vi "ProgramDevice.vi"(1 "Firmware file":path) -> ()   [LabVIEW 2010]
panel:
  out "Array 4":u32[](array[numeric])
  out "Array 3":u32[][](array[numeric])
  out "Array 2":T1(array[cluster])
  out "Array":i32[][](array[numeric])
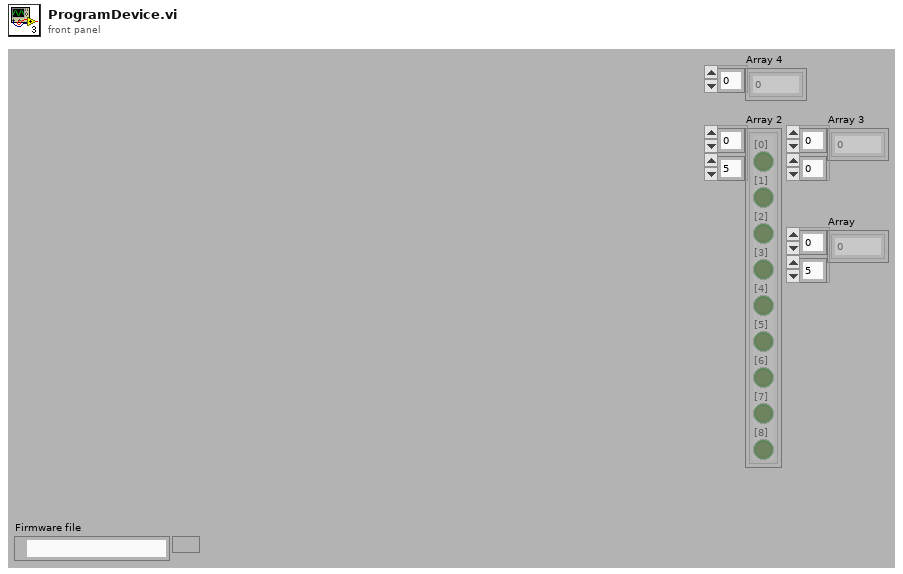
[diagram p1: front panel]
types:
  T1 = cluster{"[0]":bool, "[1]":bool, "[2]":bool, "[3]":bool, "[4]":bool, "[5]":bool, "[6]":bool, "[7]":bool, "[8]":bool}[][]
  T2 = cluster{"Clock Out MSB First":bool, "Clock Out On Positive Edge":bool}
  T3 = cluster{"Clock Pin State":bool, "Data Out Pin State":bool, "Chip Select Pin State":bool, "Chip Select Pin":u16}
  T4 = typedef "SpiDevice.ctl" = cluster{"Name":string, "Channel":string, "Location ID":u32, "Handle":u32}
  T5 = cluster{"Pin 1 State":bool, "Pin 1 Active State":bool, "Pin 2 State":bool, "Pin 2 Active State":bool, "Pin 3 State":bool, "Pin 3 Active State":bool, "Pin 4 State":bool, "Pin 4 Active State":bool, "Pin 5 State":bool, "Pin 5 Active State":bool, "Pin 6 State":bool, "Pin 6 Active State":bool, "Pin 7 State":bool, "Pin 7 Active State":bool, "Pin 8 State":bool, "Pin 8 Active State":bool}
  T6 = cluster{"Wait Data Write Complete":bool, "Wait Data Write Pin":u16, "Data Write Complete State":bool, "Data Write Timeout (ms)":u32}
  T7 = cluster{"[0]":bool, "[1]":bool, "[2]":bool, "[3]":bool, "[4]":bool, "[5]":bool, "[6]":bool, "[7]":bool, "[8]":bool}
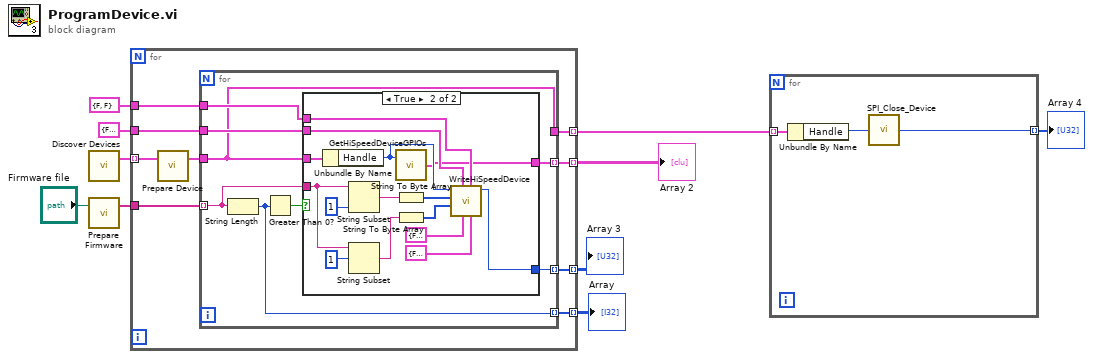
[diagram p0: block diagram]
diagram:
  n1 = call "Discover Devices.vi"() -> ("Devices"=w8:T4[])  [unwired: 2 in, 1 out]
  n2 = call "Prepare Firmware.vi"("Firmware file"="Firmware file") -> ("Firmware data"=w9:string[])  [unwired: 1 in, 1 out]
  n3 = for {
    tunnel: w9 -> [w17]
    tunnel: w8 -> [w19] mode=indexing
    tunnel: T3 {"Clock Pin State"=FALSE, "Data Out Pin State"=FALSE, "Chip Select Pin State"=FALSE, "Chip Select Pin"=0} ("Init Condition") -> [w16]
    tunnel: T2 {"Clock Out MSB First"=FALSE, "Clock Out On Positive Edge"=FALSE} ("Data Control") -> [w15]
    tunnel: [w14] -> w5 mode=indexing
    tunnel: [w13] -> w4 mode=indexing
    tunnel: [w12] -> w3 mode=indexing
    tunnel: [w11] -> w2 mode=indexing
    n4 = call "Prepare Device.vi"("SPI Device"=w19) -> ("SPI Device"=w18:T4)  [unwired: 2 in]
    n5 = for {
      tunnel: w18 -> [w20]
      tunnel: w17 -> [w25] mode=indexing
      tunnel: w16 -> [w27]
      tunnel: w15 -> [w26]
      tunnel: [w23] -> w14 mode=indexing
      tunnel: [w22] -> w13 mode=indexing
      tunnel: [w21] -> w12 mode=indexing
      tunnel: [w20] -> w11
      n6 = String Length(string=w25) -> (length=w23:i32)
      n7 = Greater Than 0?(x=w23) -> (x > 0?=w24:bool)
      n8 = case shown="True" w24 {
        tunnel: w27 -> [_ w42]
        tunnel: w26 -> [_ w41]
        tunnel: w25 -> [_ w36]
        tunnel: w20 -> [_ w31]
        tunnel: [_ w29] -> w22
        tunnel: [_ w28] -> w21
        frame False {
        }
        frame True {
          n9 = Unbundle By Name(w31) -> ("Handle"=w30:u32)
          n10 = String Subset(string=w36, length (rest)=1 ("length (rest)")) -> (substring=w39:string)  [unwired: 1 in]
          n11 = String Subset(string=w36, offset (0)=1 ("length (rest)")) -> (substring=w37:string)  [unwired: 1 in]
          n12 = call "GetHiSpeedDeviceGPIOs.vi"("Handle"=w30) -> ("High IO Values"=w29:T7)  [unwired: 1 in, 2 out]
          n13 = String To Byte Array(string=w39) -> (unsigned byte array=w38:u8[])
          n14 = String To Byte Array(string=w37) -> (unsigned byte array=w34:u8[])
          n15 = call "WriteHiSpeedDevice.vi"("High Output Pins"=T5 {"Pin 1 State"=FALSE, "Pin 1 Active State"=FALSE, "Pin 2 State"=FALSE, "Pin 2 Active State"=FALSE, "Pin 3 State"=FALSE, "Pin 3 Active State"=FALSE, "Pin 4 State"=FALSE, "Pin 4 Active State"=FALSE, "Pin 5 State"=FALSE, "Pin 5 Active State"=FALSE, "Pin 6 State"=FALSE, "Pin 6 Active State"=FALSE, "Pin 7 State"=FALSE, "Pin 7 Active State"=FALSE, "Pin 8 State"=FALSE, "Pin 8 Active State"=FALSE}, "Data Control"=w41, "Wait Data Write"=T6 {"Wait Data Write Complete"=FALSE, "Wait Data Write Pin"=0, "Data Write Complete State"=FALSE, "Data Write Timeout (ms)"=0}, "Init Condition"=w42, "Data Buffer"=w34, "Control Buffer"=w38, "Handle"=w30) -> ("Result"=w28:u32)  [unwired: 3 in, 1 out]
        }
      }
    }
  }
  "Array" <- w5
  "Array 2" <- w4
  "Array 3" <- w3
  n16 = for {
    tunnel: w2 -> [w45] mode=indexing
    tunnel: [w43] -> w1 mode=indexing
    n17 = Unbundle By Name(w45) -> ("Handle"=w44:u32)
    n18 = call "SPI_Close_Device.vi"("Handle"=w44) -> ("FTC_Status"=w43:u32)
  }
  "Array 4" <- w1
